vi "Obst Enum.vi"(1 "Obstacle Side":T1(ring), 2 "If Obstacle":T1(ring), 3 "Command":T1(ring)=enum."Back") -> (0 "Out":T1(ring))   [LabVIEW 2015]
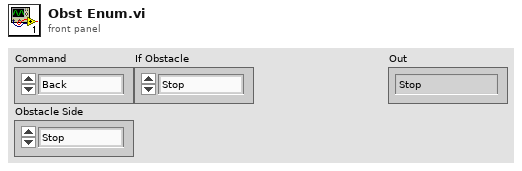
[diagram p1: front panel]
types:
  T1 = enum16{"Stop", "LED", "Front", "Back", "Left", "Right"}
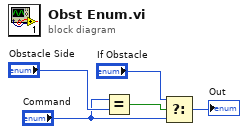
[diagram p0: block diagram]
diagram:
  n1 = Equal?(x="Command", y="Obstacle Side") -> (x = y?=w4:bool)
  n2 = Select(t="If Obstacle", s=w4, f="Command") -> (s? t:f=→"Out":T1)
